vi "Pocess Fit.vi"(8 "error in (no error)":errorcluster, 9 "Plot in":cluster{dbl[], dbl[]}[](array[cluster]), 10 "Result in":refnum<class "Acquired Result.lvclass">, 11 "Format Resonances in":refnum<class "Format Resonances.lvclass">) -> (0 "error out":errorcluster, 1 "Plot out":cluster{dbl[], dbl[]}[](array[cluster]), 2 "Result out":refnum<class "Acquired Result.lvclass">, 3 "Format Resonances out":refnum<class "Format Resonances.lvclass">)   [LabVIEW 2018, in "Format Resonances.lvclass"]
uses:
  Format Resonances.lvclass
  NHMFL_Core/Libraries/Instruments/Results/Acquired Result/Acquired Result.lvclass
  Read Elastic Moduli Configuration.vi
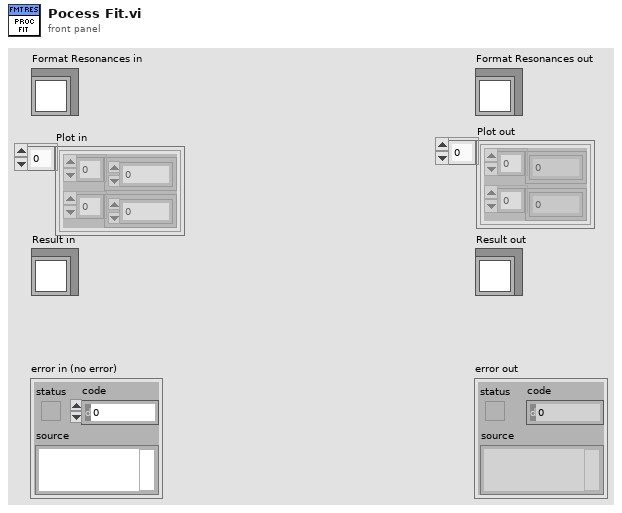
[diagram p1: front panel]
types:
  T1 = enum16{"open", "open or create", "create or replace", "create", "open (read-only)"}
  T2 = typedef "Format Resonances Configuration.ctl" = cluster{"Output header ":string, "rusin\n.dat":enum16{"NONE", "With header", "Without header"}, "Resonance detector module name":string, "Save sp*.dat":bool}
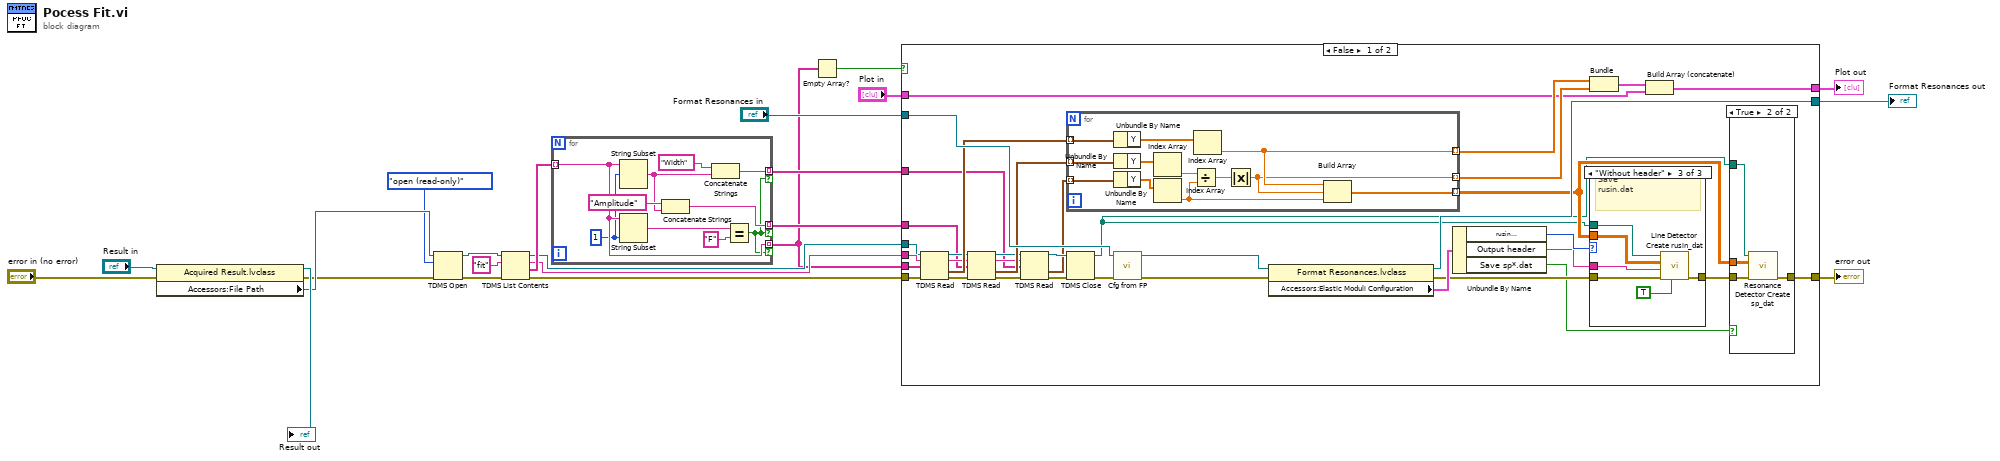
[diagram p0: block diagram]
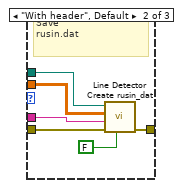
[diagram p4: hidden frame]
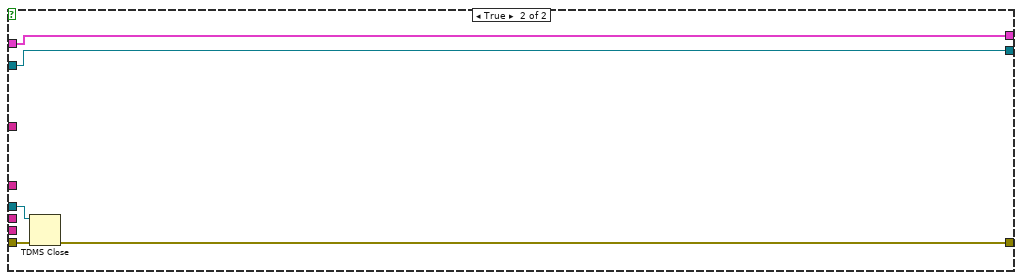
[diagram p5: hidden frame]
diagram:
  n1 = property class="Acquired Result.lvclass"(reference="Result in", error in="error in (no error)") -> (reference out=→"Result out":refnum<class "Acquired Result.lvclass">, error out=w17:errorcluster, "Accessors:File Path"=w18:path)
  n2 = TDMS Open(8:w17, 10:T1."open (read-only)" ("operation (0:open)"), 11:w18) -> (0:w14:errorcluster, 3:w15:refnum<k34>)  [unwired: 4 in]
  n3 = TDMS List Contents(4:w14, 6:"fit" ("group name"), 7:w15) -> (0:w9:errorcluster, 1:w11:string[], 2:w10:string, 3:w8:refnum<k34>)
  n4 = for {
    tunnel: w11 -> [w30] mode=indexing
    tunnel: [w30] -> w5 mode=indexing if=w23
    tunnel: [w27] -> w7 mode=indexing if=w23
    tunnel: [w24] -> w6 mode=indexing if=w23
    w29 = 1 ("length (rest)")
    n5 = String Subset(string=w30, offset (0)=w29) -> (substring=w25:string)  [unwired: 1 in]
    n6 = String Subset(string=w30, length (rest)=w29) -> (substring=w32:string)  [unwired: 1 in]
    n7 = Concatenate Strings("Amplitude" ("y"), w25) -> (w27:string)
    n8 = Concatenate Strings("Width" ("y"), w25) -> (w24:string)
    n9 = Equal?(x=w32, y="F") -> (x = y?=w23:bool)
  }
  n10 = Empty Array?(array=w5) -> (empty?=w3:bool)
  n11 = case shown="False" w3 {
    tunnel: [w68 w103] -> w22
    tunnel: "Format Resonances in" -> [w67 w103]
    tunnel: w10 -> [w65 _]
    tunnel: w9 -> [w63 w101]
    tunnel: w8 -> [w62 w100]
    tunnel: w7 -> [w58 _]
    tunnel: w6 -> [w48 _]
    tunnel: w5 -> [w46 _]
    tunnel: [w36 w99] -> w4
    tunnel: "Plot in" -> [w39 w102]
    tunnel: [w38 w102] -> w1
    frame False {
      n12 = TDMS Read(0:w62, 5:w65, 7:w46, 11:w63) -> (4:w61:refnum<k34>, 6:w60:string, 10:w64:waveform(dbl)[], 15:w59:errorcluster)  [unwired: 4 in, 2 out]
      n13 = TDMS Read(0:w61, 5:w60, 7:w58, 11:w59) -> (4:w53:refnum<k34>, 6:w49:string, 10:w57:waveform(dbl)[], 15:w52:errorcluster)  [unwired: 4 in, 2 out]
      n14 = TDMS Read(0:w53, 5:w49, 7:w48, 11:w52) -> (4:w50:refnum<k34>, 10:w47:waveform(dbl)[], 15:w51:errorcluster)  [unwired: 4 in, 3 out]
      n15 = for {
        tunnel: w64 -> [w98] mode=indexing
        tunnel: [w91] -> w56 mode=indexing
        tunnel: w57 -> [w96] mode=indexing
        tunnel: [w87] -> w55 mode=indexing
        tunnel: w47 -> [w95] mode=indexing
        tunnel: [w88] -> w35 mode=indexing
        n16 = Unbundle By Name(w98) -> ("Y"=w97:dbl[])
        n17 = Unbundle By Name(w96) -> ("Y"=w93:dbl[])
        n18 = Unbundle By Name(w95) -> ("Y"=w94:dbl[])
        n19 = Index Array(array=w93) -> (element=w89:dbl)  [unwired: 1 in]
        n20 = Index Array(array=w94) -> (element=w90:dbl)  [unwired: 1 in]
        n21 = Divide(x=w89, y=w90) -> (x/y=w92:dbl)
        n22 = Index Array(array=w97) -> (element=w91:dbl)  [unwired: 1 in]
        n23 = Absolute Value(x=w92) -> (abs(x)=w87:dbl)
        n24 = Build Array(w91, w87, w90) -> (w88:dbl[])
      }
      n25 = TDMS Close(8:w51, 11:w50) -> (0:w66:errorcluster, 3:w34:path)
      n26 = call-dynamic "Cfg from FP.vi"("error in (no error)"=w66, "Measure Object in"=w67) -> ("error out"=w41:errorcluster, "Measure Object out"=w45:refnum<class "Format Resonances.lvclass">)  [unwired: 8 in]
      n27 = property class="Format Resonances.lvclass"(reference=w45, error in=w41) -> (reference out=w68:refnum<class "Format Resonances.lvclass">, error out=w40:errorcluster, "Accessors:Elastic Moduli Configuration"=w44:T2)
      n28 = Unbundle By Name(w44) -> ("rusin\n.dat"=w43:enum16{"NONE", "With header", "Without header"}, "Output header"=w42:string, "Save sp*.dat"=w33:bool)
      n29 = Bundle(w56, w55) -> (w54:cluster{dbl[], dbl[]})  [unwired: 1 in]
      n30 = case shown="\"Without header\"" w43 {
        tunnel: w42 -> [_ w79 w85]
        tunnel: w34 -> [_ w80 w86]
        tunnel: w40 -> [w74 w78 w84]
        tunnel: [w74 w77 w83] -> w37
        tunnel: w35 -> [_ w76 w82]
        frame "NONE" {
        }
        frame "With header", Default {
          # "Save\nrusin.dat"
          n31 = call "Line Detector Create rusin_dat.vi"("New style"=FALSE, "Error In"=w78, "header"=w79, "Fit results"=w76, "File Path Control"=w80) -> ("Error Out"=w77:errorcluster)  [unwired: 6 in]
        }
        frame "Without header" {
          # "Save\nrusin.dat"
          n32 = call "Line Detector Create rusin_dat.vi"("New style"=TRUE, "Error In"=w84, "header"=w85, "Fit results"=w82, "File Path Control"=w86) -> ("Error Out"=w83:errorcluster)  [unwired: 6 in]
        }
      }
      n33 = Build Array (concatenate)(w54, w39) -> (w38:cluster{dbl[], dbl[]}[])
      n34 = case shown="True" w33 {
        tunnel: w34 -> [_ w73]
        tunnel: w37 -> [w69 w72]
        tunnel: [w69 w71] -> w36
        tunnel: w35 -> [_ w70]
        frame False {
        }
        frame True {
          n35 = call "Resonance Detector Create sp_dat.vi"("Error In"=w72, "Fit results"=w70, "File Path Control"=w73) -> ("Error Out"=w71:errorcluster)  [unwired: 8 in]
        }
      }
    }
    frame True {
      n36 = TDMS Close(8:w101, 11:w100) -> (0:w99:errorcluster)  [unwired: 1 out]
    }
  }
  "error out" <- w4
  "Format Resonances out" <- w22
  "Plot out" <- w1
